vi "Modbus Read SGL.vi"(7 "Slave Address":u8, 8 "error in (no error)":errorcluster, 10 "Register Start Address":u16 format="%x", 11 "VISA resource in":refnum<visa-resource-name>) -> (0 "error out":errorcluster, 1 "Output data float32":sgl, 3 "VISA resource out":refnum<visa-resource-name>)   [LabVIEW 2024, in "Voegtlin_NI_SMART_Modbus_Drivers.lvlib"]
doc: "Lese einen float32-Wert an der angegebenen Startadresse des selektierten Geraetes aus.\nDer COM-Port muss dazu initialisiert sein (benutze\" Modbus Init.vi\")."
uses:
  Voegtlin_NI_SMART_Modbus_Drivers.lvlib
  Enums/Modbus Comm.ctl
panel:
  out "Read register data\n U16 (array)":u16[](array[numeric])
  # "Input Data"
  # "Internal Data"
  # "Output Data"
  # "(Inputmaske in HEX)"
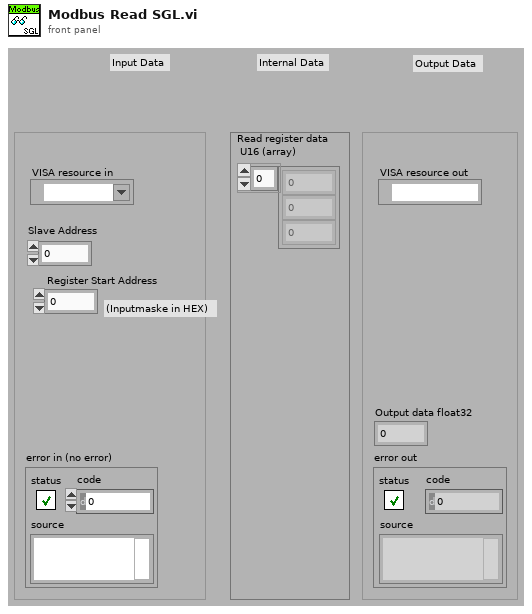
[diagram p1: front panel]
types:
  T1 = typedef "Voegtlin_NI_SMART_Modbus_Drivers.lvlib/Modbus Comm.ctl" = enum16{"Init", "Read", "Write", "Exit"}
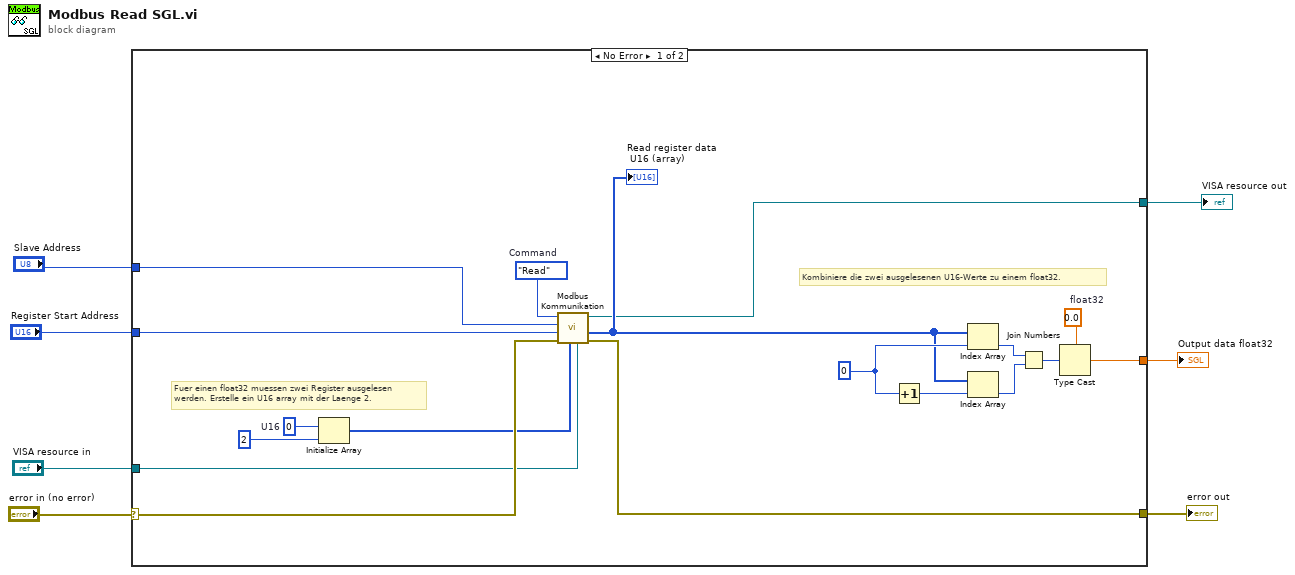
[diagram p0: block diagram]
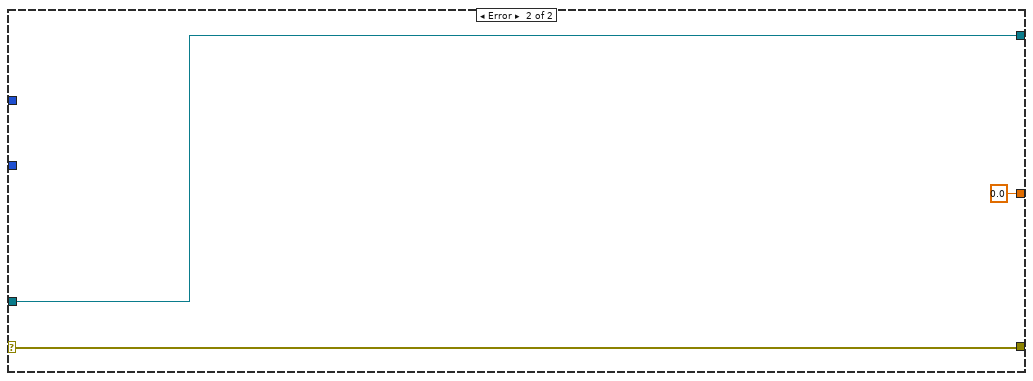
[diagram p2: hidden frame]
diagram:
  n1 = case shown="No Error" "error in (no error)" {
    selector: "error in (no error)" -> [w14 w27]
    tunnel: "Register Start Address" -> [w11 _]
    tunnel: [w13 w27] -> w4
    tunnel: [w15 sgl 0.0 ("float32")] -> w6
    tunnel: "Slave Address" -> [w10 _]
    tunnel: "VISA resource in" -> [w9 w26]
    tunnel: [w8 w26] -> w1
    frame No Error {
      w19 = sgl 0.0  # float32
      w17 = 0 ("x")
      w24 = u16 0  # U16
      w25 = Modbus_Comm."Read"  # Command
      # "Kombiniere die zwei ausgelesenen U16-Werte zu einem float32."
      # "Fuer einen float32 muessen zwei Register ausgelesen werden. Erstelle ein U16 array mit der Laenge 2."
      n2 = Initialize Array(w24, 2) -> (w12:u16[])
      n3 = call "Modbus Kommunikation.vi"("VISA resource in"=w9, "Data In / #Reads [U16]"=w12, "error in (no error)"=w14, "Register Start Address"=w11, "Slave Address"=w10, "Command"=w25) -> ("error out"=w13:errorcluster, "Data Out [U16]"=w16:u16[], "VISA resource out"=w8:refnum<visa-resource-name>)  [unwired: 3 in]
      "Read register data\n U16 (array)" <- w16
      n4 = Increment(x=w17) -> (x+1=w22:i32)
      n5 = Index Array(array=w16, index=w17) -> (element=w21:u16)
      n6 = Index Array(array=w16, index=w22) -> (element=w20:u16)
      n7 = Join Numbers(hi=w21, lo=w20) -> ((hi.lo)=w18:u32)
      n8 = Type Cast(type=w19, x=w18) -> (*(type *) &x=w15:sgl)
    }
    frame Error {
    }
  }
  "error out" <- w4
  "Output data float32" <- w6
  "VISA resource out" <- w1
